vi "WSVCAP SHL Host LL SPI Convert Channel Bytes to Bit Array.vi"(0 "SPI Data [DUT Ordered]":u8[][](array[numeric]) format="%02x", 7 "Cycle CMD Lengths Out (bits)":u8[](array[numeric]), 9 "Cycle CMD Delay Out (ticks)":u32[](array[numeric])) -> (4 "Write Data":u64[](array[numeric]) format="%016x")   [LabVIEW 2012]
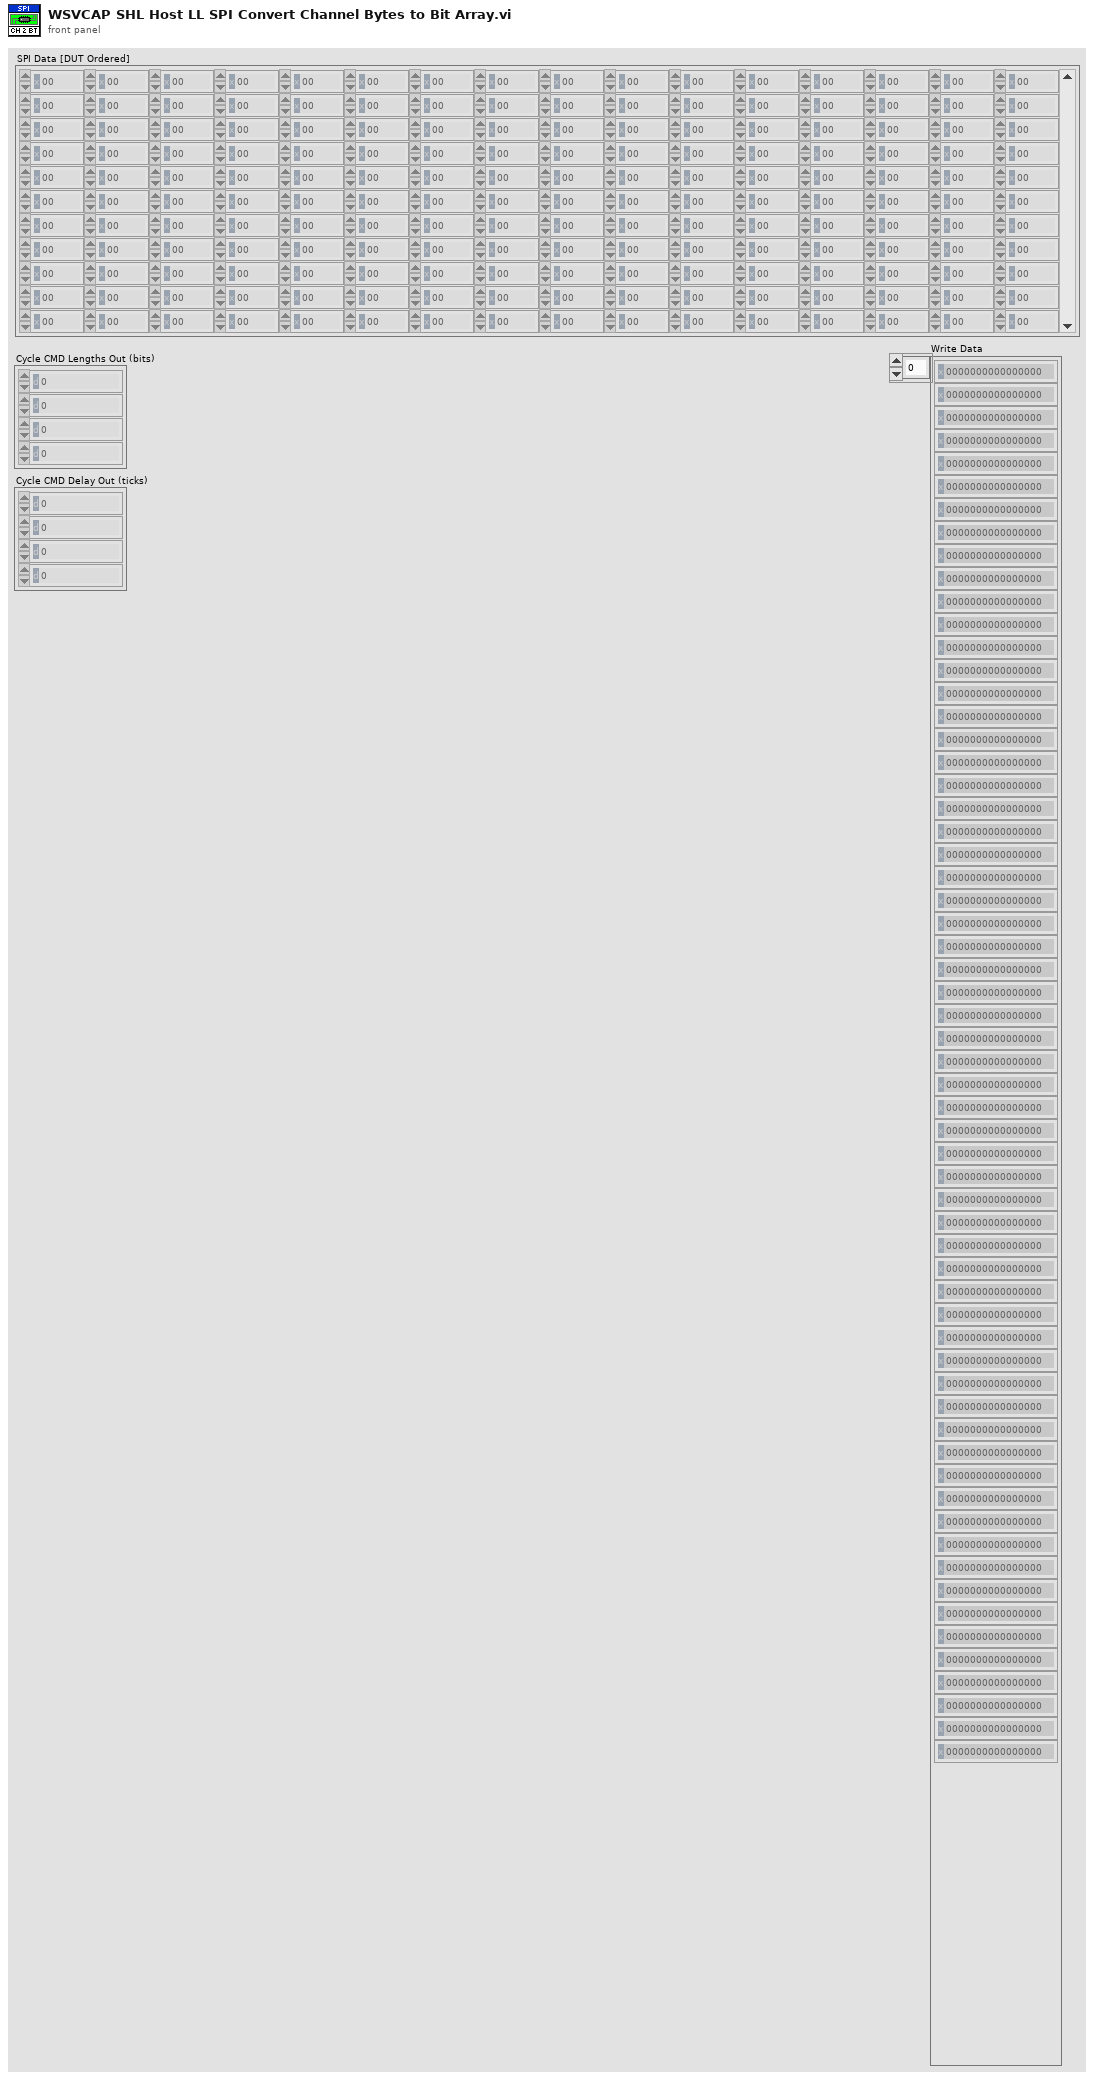
[diagram p1: front panel]
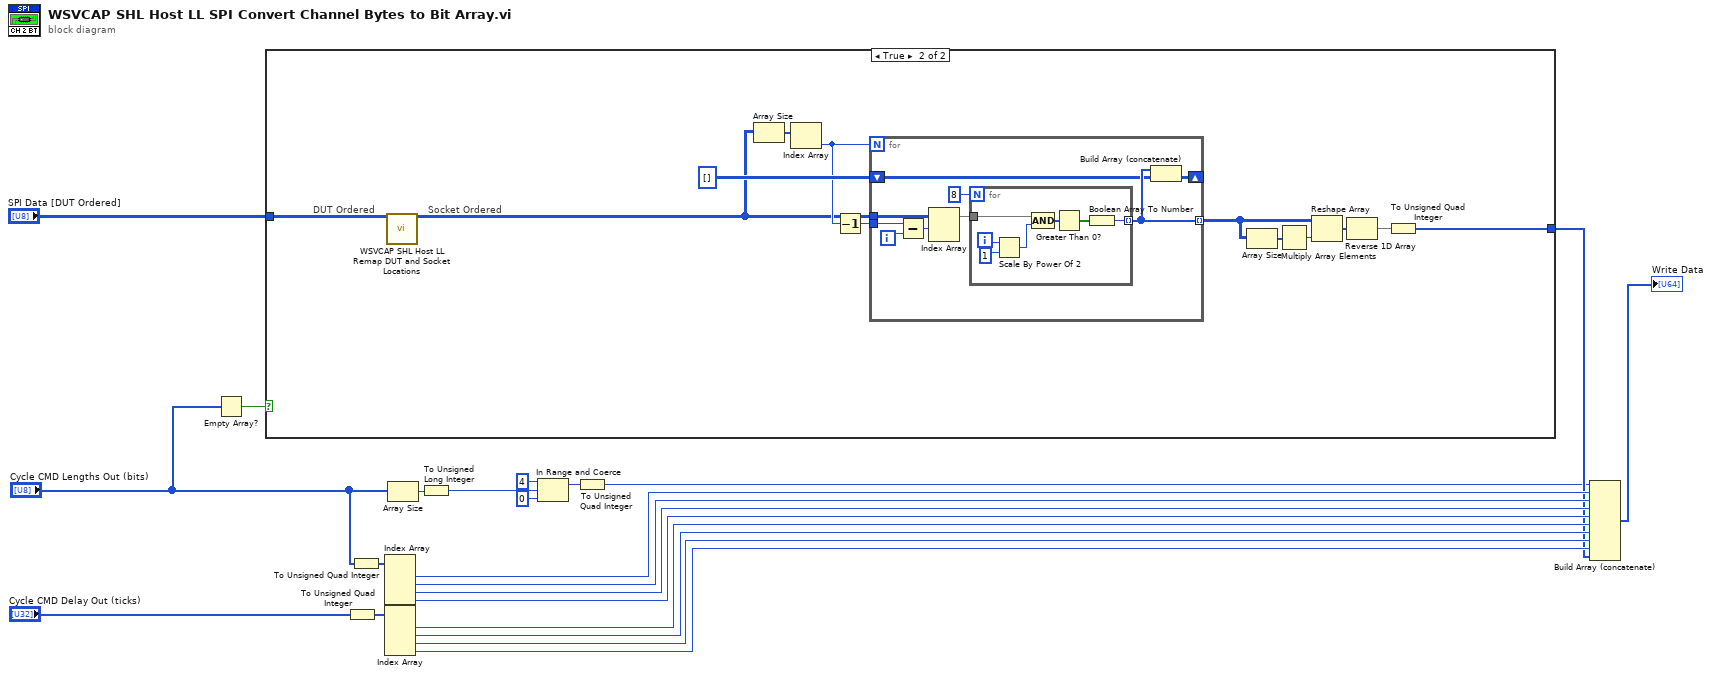
[diagram p0: block diagram]
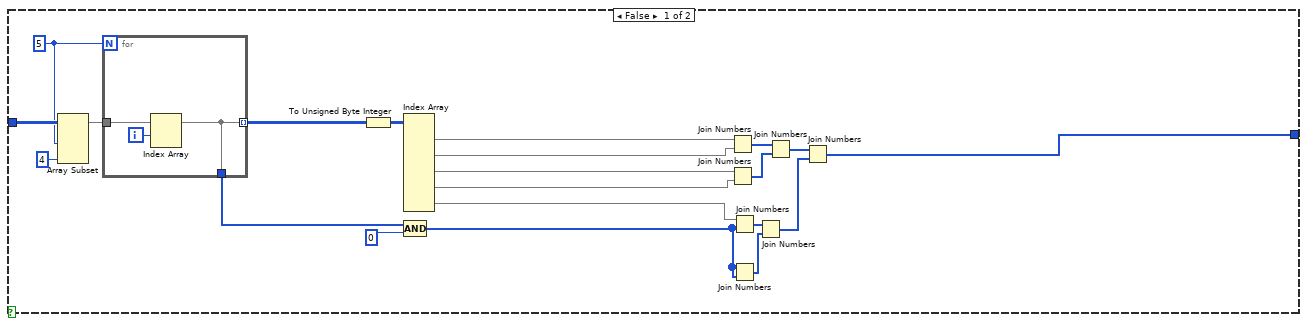
[diagram p2: hidden frame]
diagram:
  n1 = Empty Array?(array="Cycle CMD Lengths Out (bits)") -> (empty?=w3:bool)
  n2 = case shown="True" w3 {
    tunnel: "SPI Data [DUT Ordered]" -> [w29 w48]
    tunnel: [w36 w49] -> w5
    frame False {
      w27 = 5
      n3 = Array Subset(array=w29, length (row)=w27, length (col)=4 ("length")) -> (w28:u8[][])  [unwired: 2 in]
      n4 = for {
        N: w27 -> [_]
        tunnel: w28 -> [w46]
        tunnel: [w44] -> w30 mode=indexing
        tunnel: [w44] -> w25
        i -> [w45]
        n5 = Index Array(array=w46, index (row)=w45) -> (element=w44:u8[])  [unwired: 1 in]
      }
      n6 = To Unsigned Byte Integer(number=w30) -> (unsigned 8bit integer=w35:u8[][])
      n7 = Index Array(array=w35) -> (element #1=w43:u8[], element #2=w42:u8[], element #3=w41:u8[], element #4=w40:u8[], element #5=w34:u8[])  [unwired: 10 in]
      n8 = Compound Arithmetic op=AND(w25, u8 0 ("Read Data")) -> (w24:u8[])
      n9 = Join Numbers(hi=w43, lo=w42) -> ((hi.lo)=w39:u16[])
      n10 = Join Numbers(hi=w41, lo=w40) -> ((hi.lo)=w38:u16[])
      n11 = Join Numbers(hi=w34, lo=w24) -> ((hi.lo)=w33:u16[])
      n12 = Join Numbers(hi=w24, lo=w24) -> ((hi.lo)=w32:u16[])
      n13 = Join Numbers(hi=w33, lo=w32) -> ((hi.lo)=w31:u32[])
      n14 = Join Numbers(hi=w39, lo=w38) -> ((hi.lo)=w37:u32[])
      n15 = Join Numbers(hi=w37, lo=w31) -> ((hi.lo)=w36:u64[])
    }
    frame True {
      # "Socket Ordered"
      # "DUT Ordered"
      n16 = call "WSVCAP SHL Host LL Remap DUT and Socket Locations.vi"("C1 DUT Ordered Data In"=w48) -> ("C1 Socket Ordered Data Out"=w47:u8[][])  [unwired: 13 in, 5 out]
      n17 = Array Size(array=w47) -> (size(s)=w54:i32[])
      n18 = Index Array(array=w54) -> (element=w52:i32)  [unwired: 1 in]
      n19 = Decrement(x=w52) -> (x-1=w51:i32)
      n20 = for {
        N: w52 -> [_]
        tunnel: w47 -> [w63]
        tunnel: [w66] -> w58 mode=indexing
        shift-right: [w65] -> _
        shift-left: u32[][] [] -> [w64]
        tunnel: w51 -> [w59]
        i -> [w61]
        n21 = Subtract(x=w59, y=w61) -> (x-y=w60:i32)
        n22 = Index Array(array=w63, index (row)=w60) -> (element=w62:u8[])  [unwired: 1 in]
        n23 = for {
          N: 8 -> [_]
          tunnel: w62 -> [w70]
          tunnel: [w69] -> w66 mode=indexing
          i -> [w72]
          n24 = Scale By Power Of 2(n=w72, x=u8 1) -> (x*2^n=w73:u8)
          n25 = Compound Arithmetic op=AND(w70, w73) -> (w74:u8[])
          n26 = Greater Than 0?(x=w74) -> (x > 0?=w68:bool[])
          n27 = Boolean Array To Number(Boolean array=w68) -> (number=w69:u32)
        }
        n28 = Build Array (concatenate)(w66, w64) -> (w65:u32[][])
      }
      n29 = Array Size(array=w58) -> (size(s)=w57:i32[])
      n30 = Multiply Array Elements(1:w57) -> (0:w56:i32)
      n31 = Reshape Array(w58, w56) -> (w53:u32[])
      n32 = Reverse 1D Array(array=w53) -> (reversed array=w50:u32[])
      n33 = To Unsigned Quad Integer(1:w50) -> (0:w49:u64[])
    }
  }
  n34 = To Unsigned Quad Integer(1:"Cycle CMD Delay Out (ticks)") -> (0:w2:u64[])
  n35 = To Unsigned Quad Integer(1:"Cycle CMD Lengths Out (bits)") -> (0:w14:u64[])
  n36 = Index Array(array=w14) -> (element #1=w16:u64, element #2=w15:u64, element #3=w13:u64, element #4=w12:u64)  [unwired: 4 in]
  n37 = Index Array(array=w2) -> (element #1=w11:u64, element #2=w10:u64, element #3=w9:u64, element #4=w8:u64)  [unwired: 4 in]
  n38 = Array Size(array="Cycle CMD Lengths Out (bits)") -> (size(s)=w21:i32)
  n39 = To Unsigned Long Integer(number=w21) -> (unsigned 32bit integer=w6:u32)
  n40 = In Range and Coerce(upper limit=u32 4, x=w6, lower limit=u32 0) -> (coerced(x)=w18:u32)  [unwired: 1 out]
  n41 = To Unsigned Quad Integer(1:w18) -> (0:w1:u64)
  n42 = Build Array (concatenate)(w1, w16, w15, w13, w12, w11, w10, w9, w8, w5) -> (→"Write Data":u64[])
